vi "test.vi"() -> ()   [LabVIEW 2015]
panel:
  in  "Slide":dbl(slide) scale=0.0..10.0
  out "x+y":dbl
  in  "Numeric 2":dbl
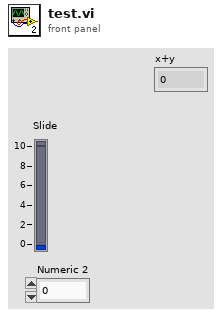
[diagram p1: front panel]
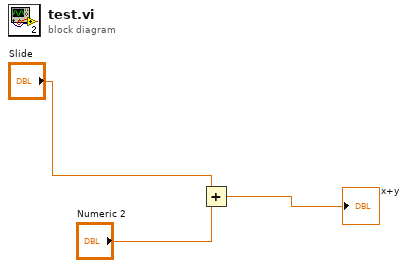
[diagram p0: block diagram]
diagram:
  n1 = Add(x="Numeric 2", y="Slide") -> (x+y=→"x+y":dbl)
